vi "Vison Save Temple.vi"(0 "Enable":bool=TRUE caption="启用", 5 "error in (no error)":errorcluster caption="错误输入（无错误）") -> (17 "创建模板程序":string, 18 "确定":bool, 19 "error out":errorcluster caption="错误输出")   [LabVIEW 2017]
doc: "显示标准对话框，提示用户输入用户名、密码等信息。\n--------------------\n\n该Express VI配置如下:\n\n显示给用户的信息:\n该输入为: \n文本输入框: 创建模板程序"
uses:
  Global System.vi
panel:
  in  "创建模板程序":string(combo)="potteryTemplete"
  out "String":string caption="字符串"
  in  "Cancel":bool caption="取消"
  in  "OK2":bool
  in  "OK1":bool
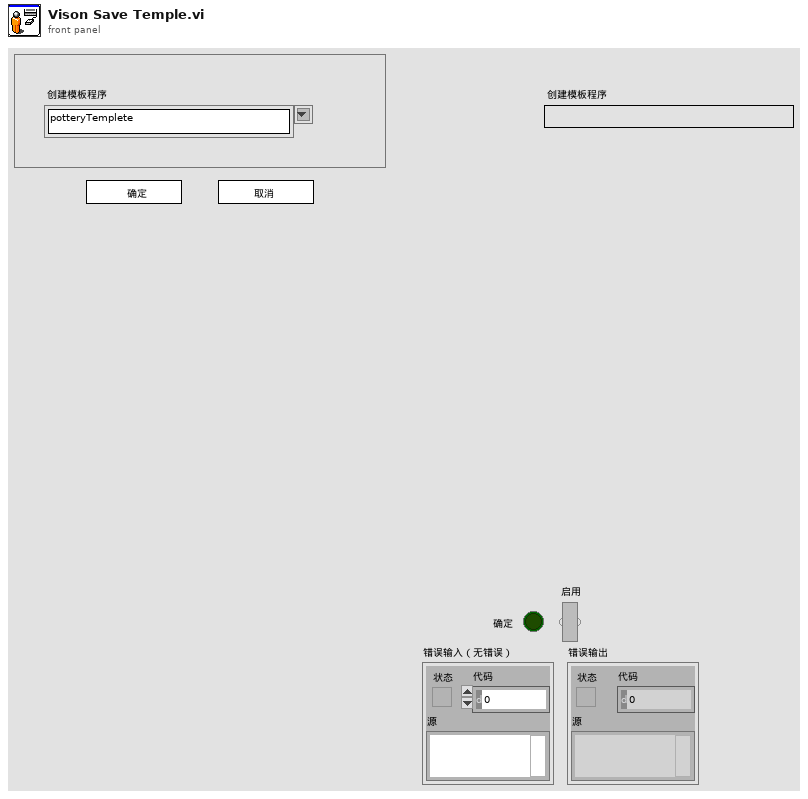
[diagram p1: front panel]
types:
  T1 = cluster{"Input Name":string, "Input Data Type":i32}[]
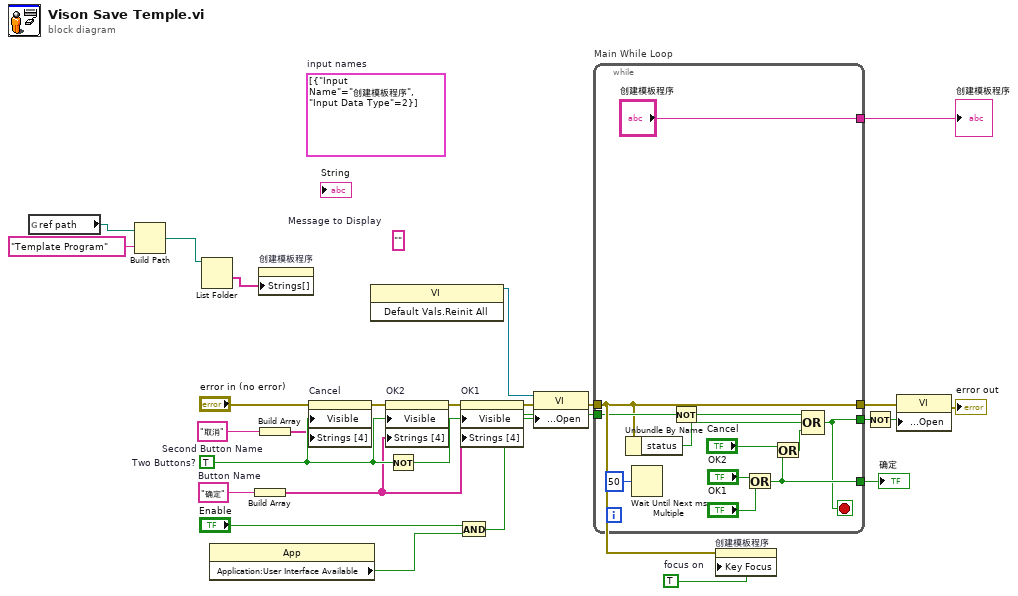
[diagram p0: block diagram]
diagram:
  w5 = TRUE  # focus on
  (unwired) T1 [{"Input Name"="创建模板程序", "Input Data Type"=2}]  # input names
  w18 = "取消"  # Second Button Name
  w16 = "确定"  # Button Name
  (unwired) ""  # Message to Display
  w26 = TRUE  # Two Buttons?
  n1 = global read "Global System.vi" "ref path"() -> (w4:path)
  n2 = Build Path(base path=w4, name or relative path="Template Program" ("名称或相对路径")) -> (appended path=w2:path)
  n3 = List Folder(path=w2) -> (folder names=w1:string[])  [unwired: 3 in, 3 out]
  n4 = property class="App"() -> ("Application:User Interface Available"=w8:bool)  [unwired: 2 in, 2 out]
  n5 = Build Array(w16) -> (w17:string[])
  n6 = property on="创建模板程序" class="CmbBox"("Strings[]"=w1) -> ()  [unwired: 2 in, 2 out]
  n7 = Build Array(w18) -> (w19:string[])
  n8 = property on="Cancel" class="Bool"(error in="error in (no error)", "Visible"=w26, "Strings [4]"=w19) -> (error out=w23:errorcluster)  [unwired: 1 in, 1 out]
  n9 = invoke class="VI" method="Default Vals.Reinit All"() -> (reference out=w7:refnum<vi>)  [unwired: 3 in, 2 out]
  n10 = property on="OK2" class="Bool"(error in=w23, "Visible"=w26, "Strings [4]"=w17) -> (error out=w22:errorcluster)  [unwired: 1 in, 1 out]
  n11 = Not(x=w26) -> (.not. x?=w24:bool)
  n12 = And(x="Enable", y=w8) -> (x .and. y?=w9:bool)
  n13 = property on="OK1" class="Bool"(error in=w22, "Visible"=w24, "Strings [4]"=w17) -> (error out=w15:errorcluster)  [unwired: 1 in, 1 out]
  n14 = property class="VI"(reference=w7, error in=w15, "Front Panel Window:Open"=w9) -> (error out=w14:errorcluster)  [unwired: 1 out]
  n15 = while "Main While Loop" {
    tunnel: [w35] -> w25
    tunnel: w9 -> [w33]
    tunnel: [w31] -> w20
    tunnel: w14 -> [w30]
    tunnel: [w30] -> w12
    tunnel: ["创建模板程序"] -> w6
    stop <- w31 stop-if-true
    n16 = Unbundle By Name(w30) -> ("status"=w28:bool)
    n17 = Wait Until Next ms Multiple(millisecond multiple=u32 50) -> ()  [unwired: 1 out]
    n18 = Not(x=w33) -> (.not. x?=w32:bool)
    n19 = Or(x="OK2", y="OK1") -> (x .or. y?=w35:bool)
    n20 = Or(x="Cancel", y=w35) -> (x .or. y?=w29:bool)
    n21 = Compound Arithmetic op=OR(w32, w28, w29) -> (w31:bool)
  }
  "确定" <- w25
  "创建模板程序" <- w6
  n22 = property on="创建模板程序" class="CmbBox"(error in=w14, "Key Focus"=w5) -> ()  [unwired: 1 in, 2 out]
  n23 = Not(x=w20) -> (.not. x?=w21:bool)
  n24 = property class="VI"(error in=w12, "Front Panel Window:Open"=w21) -> (error out=→"error out":errorcluster)  [unwired: 1 in, 1 out]
